vi "Write To Output Port.vi"(8 "error in (no error)":errorcluster {"code" format="%.0x"}, 10 "Data (0)":i32, 11 "VISA resource name":refnum<visa-resource-name>) -> (0 "error out":errorcluster {"code" format="%.0x"}, 3 "VISA resource name out":refnum<visa-resource-name>)   [LabVIEW 2016, in "Agilent N6700 Series.lvlib"]
doc: "Sets the output data on the digital control port when that port is configured for Digital I/O operation."
uses:
  <instrlib>/Agilent N6700 Series/Agilent N6700 Series.lvlib
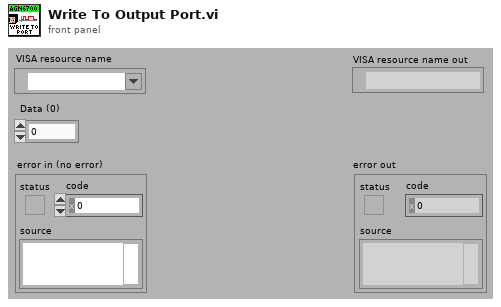
[diagram p1: front panel]
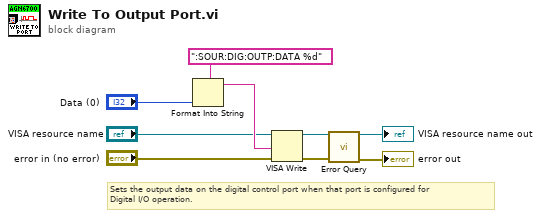
[diagram p0: block diagram]
diagram:
  # "Sets the output data on the digital control port when that port is configured for \nDigital I/O operation."
  n1 = Format Into String(format string=":SOUR:DIG:OUTP:DATA %d", "Data (0)") -> (resulting string=w8:string)  [unwired: 2 in, 1 out]
  n2 = VISA Write(VISA resource name="VISA resource name", write buffer=w8, error in (no error)="error in (no error)") -> (VISA resource name out=w2:refnum<visa-resource-name>, error out=w1:errorcluster)  [unwired: 1 out]
  n3 = call <instrlib>:"Error Query.vi"("VISA resource name"=w2, "error in (no error)"=w1) -> ("VISA resource name out"=→"VISA resource name out":refnum<visa-resource-name>, "error out"=→"error out":errorcluster)  [unwired: 10 in, 2 out]
